vi "电机定位1.1（只处理采集卡）.vi"(0 "VISA I":refnum<visa-resource-name>, 1 "等待时间(ms)":u32=40, 2 "细分设置":dbl=8.0, 3 "电机急停":bool, 4 "X":dbl, 5 "精度":dbl=0.001, 6 "pulDDR2Length":u32, 7 "量程选择":u32, 8 "hDevice":i32, 10 "M-length":dbl, 12 "N-length":dbl) -> (13 "hDevice out":i32, 14 "VISA O":refnum<visa-resource-name>, 18 "X":dbl, 19 "Y":dbl)   [LabVIEW 2016]
uses:
  <vilib>/Analysis/2dsp.llb/Real FFT.vi
  <vilib>/Utility/file.llb/Write Delimited Spreadsheet (DBL).vi
  <vilib>/Utility/file.llb/Read Delimited Spreadsheet (DBL).vi
  <vilib>/Analysis/NI_AALBase.lvlib
  <vilib>/Analysis/NI_AALPro.lvlib
panel:
  out "有效值":dbl
  out "空扫底噪":cdb[](array[numeric])
  out "采集卡底噪":cdb[](array[numeric])
  in  "保存信号":bool
  out "幅频谱":dbl[](graph)
  out "时域谱":dbl[](graph)
  in  "查询信号":bool
  in  "Y":dbl
  in  "确定":bool
  in  "ESC":bool
  # "时域谱"
  # "频域谱"
  # "目标位置"
  # "实时位置"
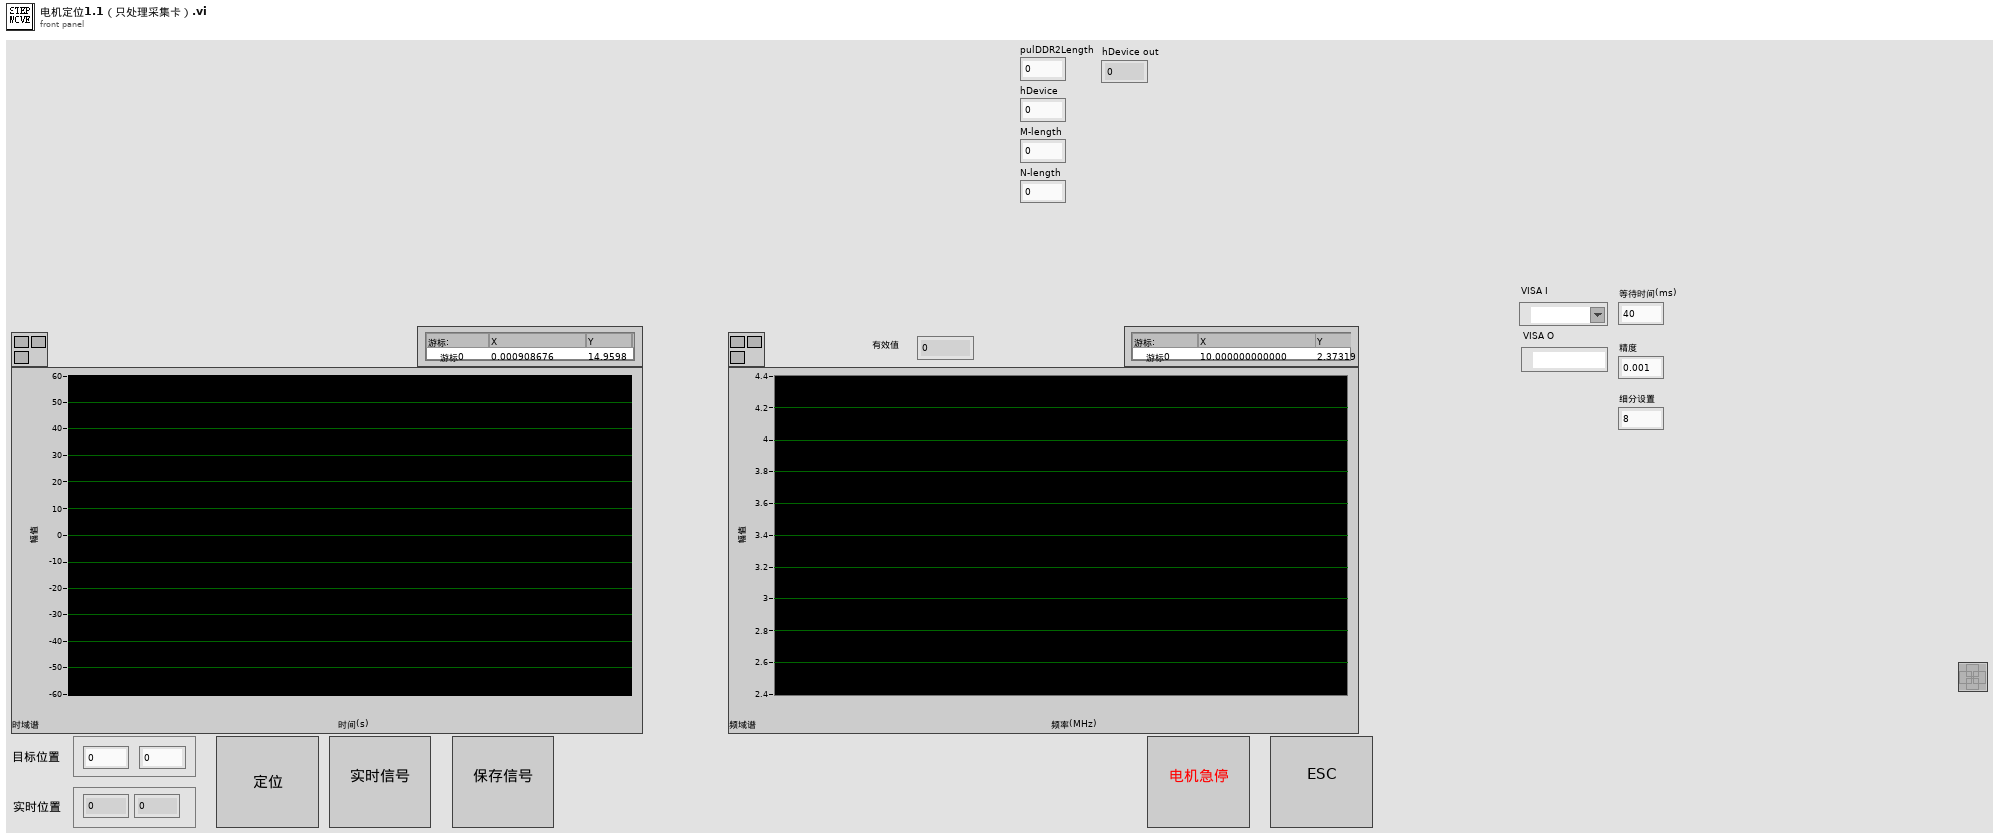
[diagram p1: front panel]
types:
  T1 = enum16{"open", "replace", "create", "open or create", "replace or create", "replace or create with confirmation"}
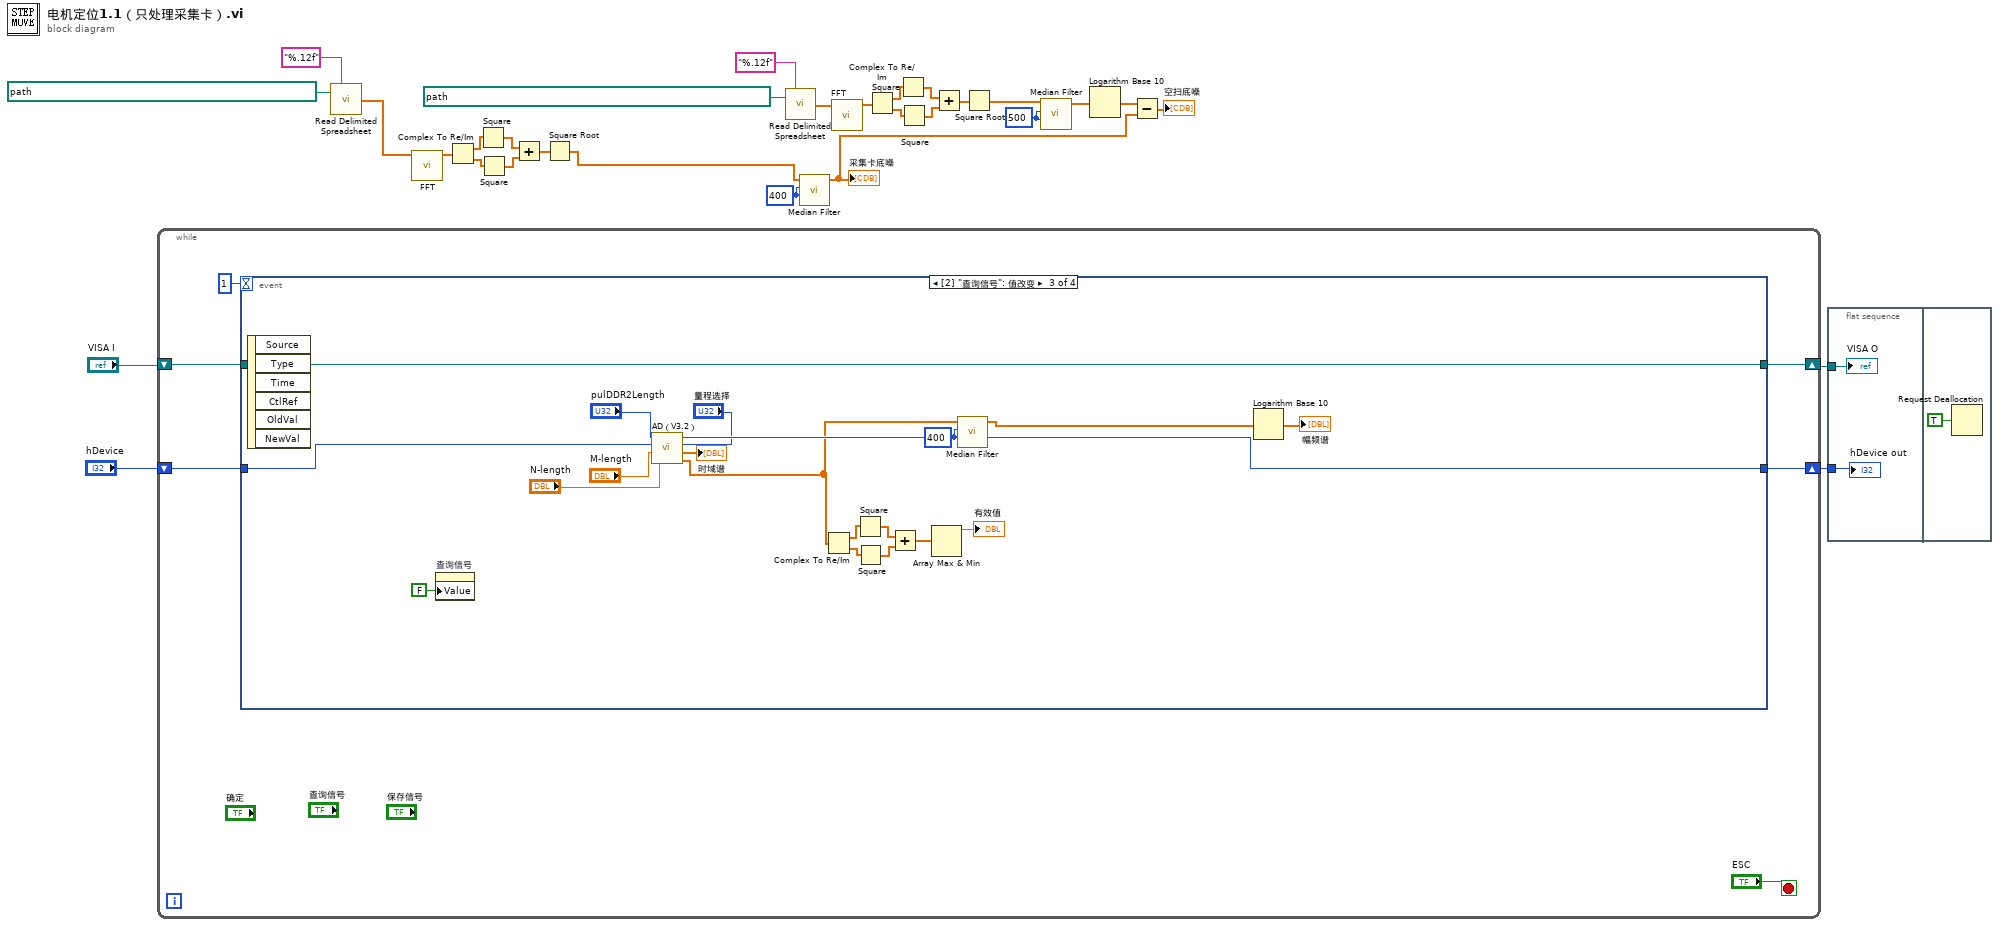
[diagram p0: block diagram]
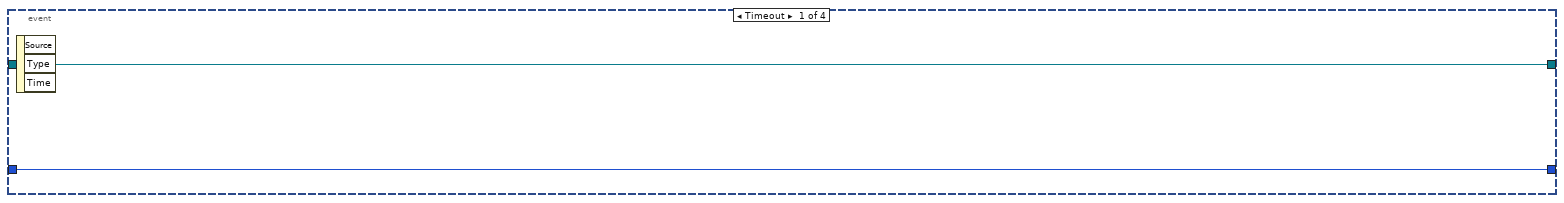
[diagram p2: hidden frame]
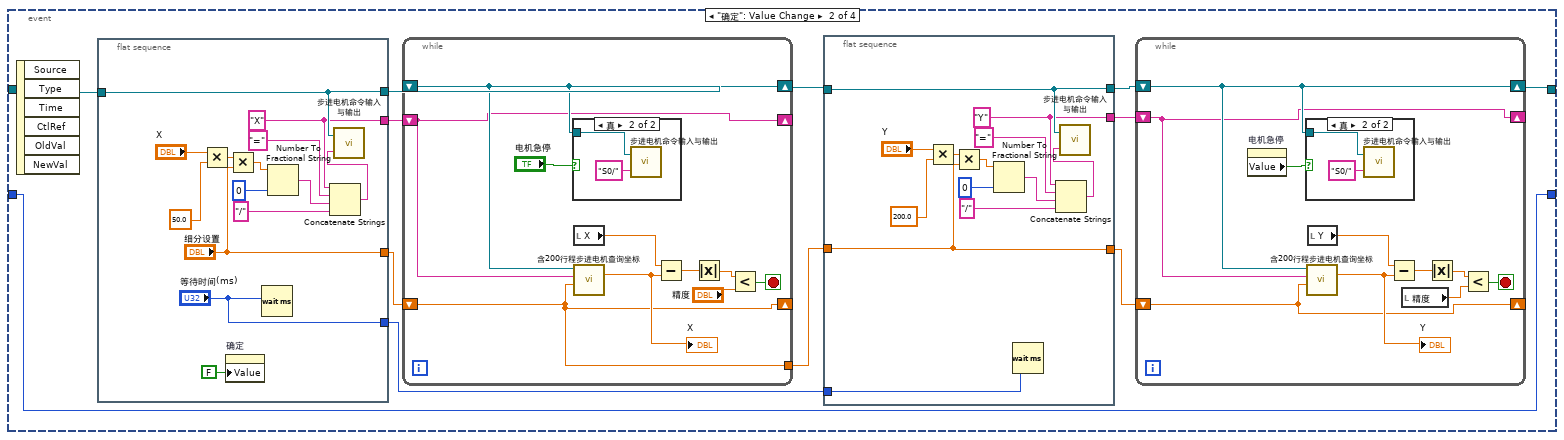
[diagram p3: hidden frame]
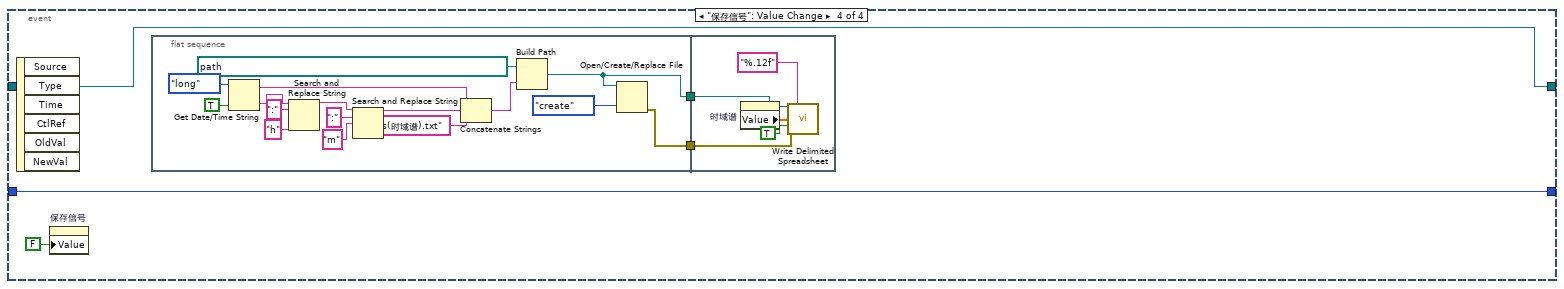
[diagram p6: hidden frame]
diagram:
  w6 = 400 ("left rank")
  w24 = 500 ("left rank")
  n1 = while {
    shift-right: [w35] -> w30
    shift-left: "VISA I" -> [w36]
    shift-right: [w32] -> w27
    shift-left: "hDevice" -> [w33]
    stop <- "ESC" stop-if-true
    n2 = event shown="[2] \"查询信号\": 值改变" {
      selector: _ -> [_ _ _ _]
      dyn-events: _ -> [_ _ _ _]
      timeout: 1 -> [_ _ _ _]
      tunnel: w36 -> [w38 w50 w120 w124]
      tunnel: [w38 w49 w120 w124] -> w35
      tunnel: w33 -> [w37 w39 w116 w123]
      tunnel: [w37 w39 w115 w123] -> w32
      event Timeout {
        n3 = event-data() -> ()  [unwired: 1 in, 3 out]
      }
      event "确定": Value Change {
        n4 = event-data() -> ()  [unwired: 1 in, 6 out]
        n5 = flat-sequence {
          tunnel: w50 -> [w93]
          tunnel: [w93] -> w48
          tunnel: ["细分设置"] -> w47
          tunnel: [w90] -> w46
          tunnel: ["等待时间(ms)"] -> w41
          frame #0 {
            w90 = "X"
            n6 = Multiply(x="X", y=50.0 ("x")) -> (x*y=w96:dbl)
            n7 = property on="确定" class="Bool (严格)"("Value"=FALSE ("确定")) -> ()  [unwired: 2 in, 2 out]
            n8 = Multiply(x=w96, y="细分设置") -> (x*y=w101:dbl)
            n9 = Wait (ms)(milliseconds to wait="等待时间(ms)") -> ()  [unwired: 1 out]
            n10 = Number To Fractional String(number=w101, precision (6)=i16 0 ("精度(6)")) -> (F-format string=w99:string)  [unwired: 2 out]
            n11 = Concatenate Strings(w90, "=" ("字符串"), w99, "/" ("字符串")) -> (w95:string)
            n12 = call "步进电机命令输入与输出.vi"("输入字符串"=w95, "串口通信端口"=w93) -> ()  [unwired: 1 out]
          }
        }
        n13 = while {
          tunnel: [w76] -> w40
          shift-right: [w82] -> w42
          shift-left: w48 -> [w82]
          shift-right: [w77] -> _
          shift-left: w46 -> [w77]
          shift-right: [w76] -> _
          shift-left: w47 -> [w76]
          stop <- w85 stop-if-true
          n14 = case shown="真" "电机急停" {
            tunnel: w82 -> [_ w86]
            frame False {
            }
            frame True {
              n15 = call "步进电机命令输入与输出.vi"("输入字符串"="S0/", "串口通信端口"=w86) -> ()  [unwired: 1 out]
            }
          }
          n16 = local read "X"() -> (w80:dbl)
          n17 = call "含200行程步进电机查询坐标.vi"("细分设置"=w76, "查询坐标轴"=w77, "串口通信端口"=w82) -> ("坐标(mm)"=w79:dbl)  [unwired: 8 in]
          "X" <- w79
          n18 = Subtract(x=w80, y=w79) -> (x-y=w84:dbl)
          n19 = Absolute Value(x=w84) -> (abs(x)=w83:dbl)
          n20 = Less?(x=w83, y="精度") -> (x < y?=w85:bool)
        }
        n21 = flat-sequence {
          tunnel: w42 -> [w67]
          tunnel: [w67] -> w45
          tunnel: [w63] -> w44
          tunnel: [w65] -> w43
          tunnel: w41 -> [w64]
          tunnel: w40 -> [w63]
          frame #0 {
            w65 = "Y"
            n22 = Multiply(x="Y", y=200.0 ("x")) -> (x*y=w70:dbl)
            n23 = Multiply(x=w70, y=w63) -> (x*y=w75:dbl)
            n24 = Number To Fractional String(number=w75, precision (6)=i16 0 ("精度(6)")) -> (F-format string=w73:string)  [unwired: 2 out]
            n25 = Wait (ms)(milliseconds to wait=w64) -> ()  [unwired: 1 out]
            n26 = Concatenate Strings(w65, "=" ("字符串"), w73, "/" ("字符串")) -> (w69:string)
            n27 = call "步进电机命令输入与输出.vi"("输入字符串"=w69, "串口通信端口"=w67) -> ()  [unwired: 1 out]
          }
        }
        n28 = while {
          shift-right: [w57] -> w49
          shift-left: w45 -> [w57]
          shift-right: [w52] -> _
          shift-left: w43 -> [w52]
          shift-right: [w51] -> _
          shift-left: w44 -> [w51]
          stop <- w60 stop-if-true
          n29 = property on="电机急停" class="Bool (严格)"() -> ("Value"=w53:bool)  [unwired: 2 in, 2 out]
          n30 = case shown="真" w53 {
            tunnel: w57 -> [_ w61]
            frame False {
            }
            frame True {
              n31 = call "步进电机命令输入与输出.vi"("输入字符串"="S0/", "串口通信端口"=w61) -> ()  [unwired: 1 out]
            }
          }
          n32 = call "含200行程步进电机查询坐标.vi"("细分设置"=w51, "查询坐标轴"=w52, "串口通信端口"=w57) -> ("坐标(mm)"=w55:dbl)  [unwired: 8 in]
          "Y" <- w55
          n33 = local read "Y"() -> (w56:dbl)
          n34 = Subtract(x=w56, y=w55) -> (x-y=w59:dbl)
          n35 = local read "精度"() -> (w54:dbl)
          n36 = Absolute Value(x=w59) -> (abs(x)=w58:dbl)
          n37 = Less?(x=w58, y=w54) -> (x < y?=w60:bool)
        }
      }
      event "查询信号": Value Change {
        w107 = 400 ("left rank")
        n38 = event-data() -> ()  [unwired: 1 in, 6 out]
        n39 = property on="查询信号" class="Bool (严格)"("Value"=FALSE ("查询信号")) -> ()  [unwired: 2 in, 2 out]
        n40 = call "AD（V3.2）.vi"("量程选择"="量程选择", "N-length"="N-length", "M-length"="M-length", "hDevice"=w116, "待读取数据长度"="pulDDR2Length") -> ("幅频谱"=w103:dbl[], "时域谱"=→"时域谱":dbl[], "hDevice out"=w115:i32)  [unwired: 4 in]
        n41 = Complex To Re/Im(x + iy=w103) -> (x=w110:dbl[], y=w111:dbl[])
        n42 = Square(x=w110) -> (x^2=w112:dbl[])
        n43 = Square(x=w111) -> (x^2=w113:dbl[])
        n44 = Add(x=w112, y=w113) -> (x+y=w109:dbl[])
        n45 = Array Max & Min(array=w109) -> (max value=→"有效值":dbl)  [unwired: 3 out]
        n46 = call <vilib>:"Median Filter.vi"("right rank"=w107, "left rank"=w107, "X"=w103) -> ("Filtered X"=w102:dbl[])  [unwired: 7 in, 1 out]
        n47 = Logarithm Base 10(1:w102) -> (0:→"幅频谱":dbl[])
      }
      event "保存信号": Value Change {
        n48 = event-data() -> ()  [unwired: 1 in, 6 out]
        n49 = property on="保存信号" class="Bool (严格)"("Value"=FALSE ("保存信号")) -> ()  [unwired: 2 in, 2 out]
        n50 = flat-sequence {
          tunnel: [w139] -> w122
          tunnel: [w138] -> w121
          tunnel: w122 -> [w143]
          tunnel: w121 -> [w142]
          frame #0 {
            n51 = Get Date/Time String(date format (0)=enum16{"short", "long", "abbreviated"}."long" ("日期格式(0)"), want seconds? (F)=TRUE ("需要秒？(F)")) -> (date string=w130:string, time string=w131:string)  [unwired: 1 in]
            n52 = Search and Replace String(input string=w131, search string=":" ("搜索字符串"), replace string="h" ("替换字符串(\"\")")) -> (result string=w136:string)  [unwired: 5 in, 3 out]
            n53 = Search and Replace String(input string=w136, search string=":" ("搜索字符串"), replace string="m" ("替换字符串(\"\")")) -> (result string=w129:string)  [unwired: 5 in, 3 out]
            n54 = Concatenate Strings(w130, w129, "s(时域谱).txt" ("字符串")) -> (w128:string)
            n55 = Build Path(base path=path "C:/Users/H301/Desktop/art采集实验数据/单点时域谱" ("基路径"), name or relative path=w128) -> (appended path=w139:path)
            n56 = Open/Create/Replace File(file path (use dialog)=w139, operation (0:open)=T1."create" ("操作(0:open)")) -> (error out=w138:errorcluster)  [unwired: 4 in, 2 out]
          }
          frame #1 {
            n57 = property on="时域谱" class="WFGraph (严格)"() -> ("Value"=w144:dbl[])  [unwired: 2 in, 2 out]
            n58 = call-poly <vilib>:"Write Delimited Spreadsheet.vi"("file path (dialog if empty)"=w143, "format (%.3f)"="%.12f", "1D data"=w144, "append to file? (new file:F)"=TRUE, "error in (no error)"=w142) -> ()  [unwired: 9 in, 2 out]
          }
        }
      }
    }
  }
  n59 = call-poly <vilib>:"Read Delimited Spreadsheet.vi"("file path (dialog if empty)"=path "C:/Users/H301/Desktop/art采集实验数据/2018年7月17日9h55m04s(采集卡底噪).txt", "format (%.3f)"="%.12f") -> ("first row"=w7:dbl[])  [unwired: 8 in, 5 out]
  n60 = call-poly <vilib>:"FFT.vi"("X"=w7) -> ("FFT {X}"=w10:cdb[])  [unwired: 9 in, 1 out]
  n61 = Complex To Re/Im(x + iy=w10) -> (x=w8:dbl[], y=w9:dbl[])
  n62 = Square(x=w8) -> (x^2=w11:dbl[])
  n63 = Square(x=w9) -> (x^2=w12:dbl[])
  n64 = Add(x=w11, y=w12) -> (x+y=w13:dbl[])
  n65 = Square Root(x=w13) -> (sqrt(x)=w1:dbl[])
  n66 = call-poly <vilib>:"Read Delimited Spreadsheet.vi"("file path (dialog if empty)"=path "C:/Users/H301/Desktop/art采集实验数据/信号源均值底噪.txt", "format (%.3f)"="%.12f") -> ("first row"=w23:dbl[])  [unwired: 8 in, 5 out]
  n67 = call <vilib>:"Median Filter.vi"("right rank"=w6, "left rank"=w6, "X"=w1) -> ("Filtered X"=w3:dbl[])  [unwired: 7 in, 1 out]
  "采集卡底噪" <- w3
  n68 = call-poly <vilib>:"FFT.vi"("X"=w23) -> ("FFT {X}"=w18:cdb[])  [unwired: 9 in, 1 out]
  n69 = Complex To Re/Im(x + iy=w18) -> (x=w20:dbl[], y=w19:dbl[])
  n70 = Square(x=w20) -> (x^2=w17:dbl[])
  n71 = Square(x=w19) -> (x^2=w16:dbl[])
  n72 = Add(x=w17, y=w16) -> (x+y=w15:dbl[])
  n73 = Square Root(x=w15) -> (sqrt(x)=w14:dbl[])
  n74 = call <vilib>:"Median Filter.vi"("right rank"=w24, "left rank"=w24, "X"=w14) -> ("Filtered X"=w5:dbl[])  [unwired: 7 in, 1 out]
  n75 = Logarithm Base 10(1:w5) -> (0:w4:dbl[])
  n76 = Subtract(x=w4, y=w3) -> (x-y=→"空扫底噪":dbl[])
  n77 = flat-sequence {
    tunnel: w30 -> [w148]
    tunnel: w27 -> [w147]
    frame #0 {
      "VISA O" <- w148
      "hDevice out" <- w147
    }
    frame #1 {
      n78 = Request Deallocation(TRUE ("标志")) -> ()
    }
  }
